vi "setLevel.vi"(6 "Output Channel":T1, 8 "error in (no error)":errorcluster, 9 "Slew (V/s)":dbl, 10 "Level (V)":dbl, 11 "Inst.RP100 in":refnum<class "Inst.RP100.lvclass">) -> (0 "error out":errorcluster, 3 "Inst.RP100 out":refnum<class "Inst.RP100.lvclass">)   [LabVIEW 2019, in "Inst.RP100.lvclass"]
doc: "Set the output <b>Level</b> with <b>Slew</b> rate on the selected <b>Output Channel</b>"
uses:
  Inst.RP100.lvclass
  Typedefs/Channel--Num.ctl
  Typedefs/Inst.RP100.Commands--Enum.ctl
  Typedefs/setLevel--Cluster.ctl
  a747f858-0bd6-4591-9409-4ed82dc3170c.vi
  a747f858-0bd6-4591-9409-4ed82dc3170c.vi/b2fc4626-9113-4d88-b8d6-aae50b62ac76.vi
  a747f858-0bd6-4591-9409-4ed82dc3170c.vi/b2fc4626-9113-4d88-b8d6-aae50b62ac76.vi/82a0d06e-8123-4040-bb49-e1c2df7066ce.vi
  a747f858-0bd6-4591-9409-4ed82dc3170c.vi/b2fc4626-9113-4d88-b8d6-aae50b62ac76.vi/1abaf707-e0d5-4be1-a8cc-a771a937af54.vi
  <vilib>/Utility/Data Type/Get Type Information.vi
  <vilib>/JDP Science/JSONtext/JSON text to Variant.vi
  <vilib>/JDP Science/JSONtext/LVClass Serializer/JSONtext LVClass Serializer.lvclass
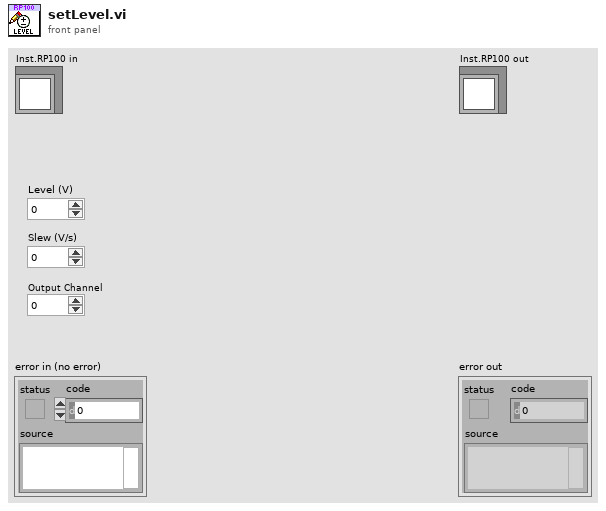
[diagram p1: front panel]
types:
  T1 = typedef "Inst.RP100.lvclass/Channel--Num.ctl" = i32
  T2 = typedef "Inst.RP100.lvclass/setLevel--Cluster.ctl" = cluster{"channel":T1, "level":dbl, "slew":dbl}
  T3 = typedef "Inst.RP100.lvclass/Inst.RP100.Commands--Enum.ctl" = enum16{"setState", "setLevel", "getLevel"}
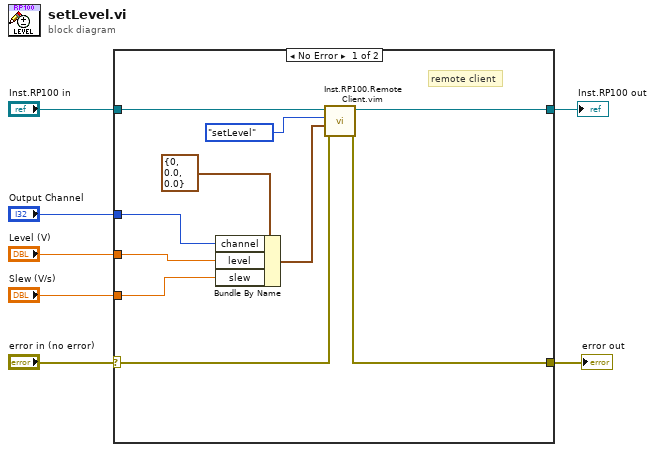
[diagram p0: block diagram]
diagram:
  n1 = case shown="No Error" "error in (no error)" {
    selector: "error in (no error)" -> [w8 w19]
    tunnel: [w15 w19] -> w6
    tunnel: "Level (V)" -> [w11 _]
    tunnel: "Inst.RP100 in" -> [w17 w18]
    tunnel: [w16 w18] -> w3
    tunnel: "Slew (V/s)" -> [w10 _]
    tunnel: "Output Channel" -> [w12 _]
    frame No Error {
      # "remote client"
      n2 = Bundle By Name(cluster=T2 {"channel"=0, "level"=0.0, "slew"=0.0} ("setLevel"), "channel"=w12, "level"=w11, "slew"=w10) -> (w9:T2)
      n3 = call "Inst.RP100.Remote Client.vim"("error in (no error)"=w8, "params"=w9, "Commands"=Inst.RP100.Commands--Enum."setLevel", "Inst.RP100 in"=w17) -> ("error out"=w15:errorcluster, "Inst.RP100 out"=w16:refnum<class "Inst.RP100.lvclass">)  [unwired: 5 in, 1 out]
    }
    frame Error {
    }
  }
  "error out" <- w6
  "Inst.RP100 out" <- w3
